vi "punto4.vi"() -> ()   [LabVIEW 2021]
panel:
  out "Led2":bool
  in  "Led2 command":bool
  out "Led1":bool
  in  "Led1 command":bool
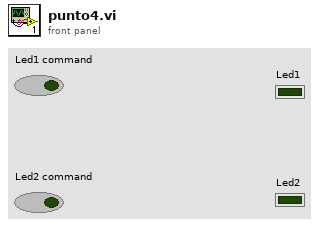
[diagram p1: front panel]
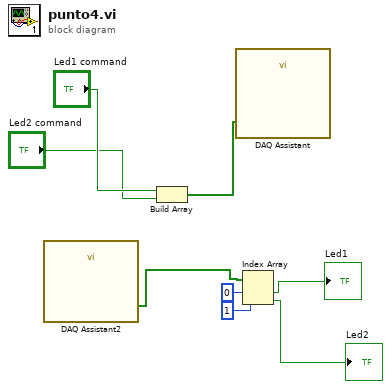
[diagram p0: block diagram]
diagram:
  n1 = call "DAQ Assistant2"() -> ("data"=w5:bool[])  [unwired: 17 in, 2 out]
  n2 = Build Array("Led1 command", "Led2 command") -> (w7:bool[])
  n3 = call "DAQ Assistant"("data"=w7) -> ()  [unwired: 17 in, 2 out]
  n4 = Index Array(array=w5, index #1=0 ("index"), index #2=1 ("index")) -> (element #1=→"Led1":bool, element #2=→"Led2":bool)
